vi "GetHelp.vi"(11 "BuildFromSource in":refnum<class "CiPipeline.lvclass">) -> (2 "Help":string, 3 "BuildFromSource out":refnum<class "CiPipeline.lvclass">)   [LabVIEW 2024, in "CiPipeline.lvclass"]
uses:
  CiPipeline.lvclass
  CiPipeline.lvclass/CiPipeline.ctl
  usr/local/natinst/nilvcli/Operations/CoreOperation/CoreOperation.lvclass
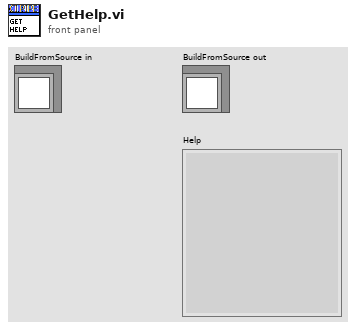
[diagram p1: front panel]
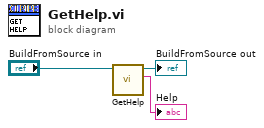
[diagram p0: block diagram]
diagram:
  n1 = call-parent "GetHelp.vi"("CoreOperation in"="BuildFromSource in") -> ("Help"=→"Help":string, "CoreOperation out"=→"BuildFromSource out":refnum<class "CiPipeline.lvclass">)  [unwired: 9 in]
